vi "Get Frequency Scale.vi"(2 "f0":dbl step=1.0, 3 "df":dbl) -> (1 "X Scale.Offset and Multiplier":T1)   [LabVIEW 2021]
uses:
  <vilib>/Utility/miscctls.llb/LVOffsetAndMultiplierTypeDef.ctl
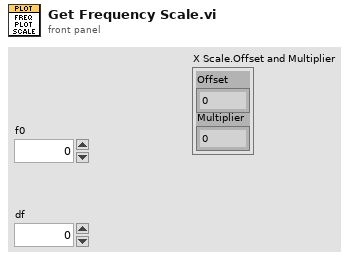
[diagram p1: front panel]
types:
  T1 = typedef "LVOffsetAndMultiplierTypeDef.ctl" = cluster{"Offset":dbl, "Multiplier":dbl}
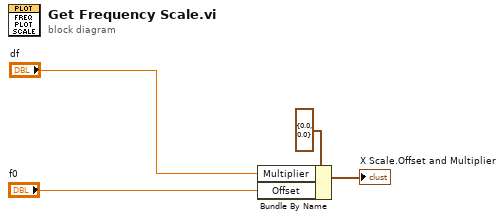
[diagram p0: block diagram]
diagram:
  n1 = Bundle By Name(cluster=T1 {"Offset"=0.0, "Multiplier"=0.0} ("X Scale.Offset and Multiplier"), "Multiplier"="df", "Offset"="f0") -> (→"X Scale.Offset and Multiplier":T1)
